vi "_text_input.vi"(9 "入力文字列":string, 11 "?":string) -> (3 "出力文字列":string)   [LabVIEW 2017]
panel:
  in  "OKボタン":bool
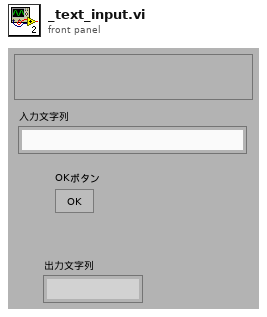
[diagram p1: front panel]
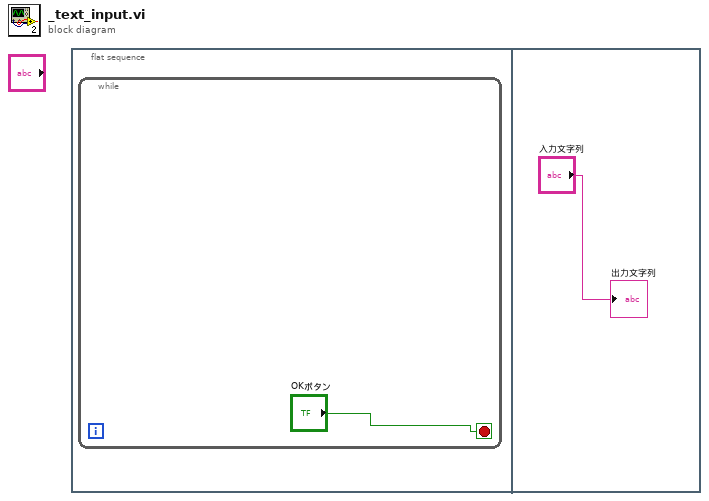
[diagram p0: block diagram]
diagram:
  n1 = flat-sequence {
    frame #0 {
      n2 = while {
        stop <- "OKボタン" stop-if-true
      }
    }
    frame #1 {
      "出力文字列" <- "入力文字列"
    }
  }
